vi "DSF.Engine.Transfer Group.Move Channels to Engine.vi"(8 "error in (no error)":errorcluster, 11 "Transfer Group in":refnum<class "DSF.Engine.Transfer Group.lvclass">) -> (0 "error out":errorcluster, 3 "Transfer Group out":refnum<class "DSF.Engine.Transfer Group.lvclass">)   [LabVIEW 2017, in "DSF.Engine.lvlib" / "DSF.Engine.Transfer Group.lvclass"]
uses:
  DSF.Engine.Transfer Group.lvclass
  DSF.Engine.Transfer Group.lvclass/DSF.Engine.Transfer Group.ctl
  DSF.Engine.Transfer.lvclass/DSF.Engine.Transfer.ctl
  DSF.Engine.Transfer.lvclass
  Built/Windows/Dependencies/Memory Manager.lvlibp/1abvi3w/vi.lib/National Instruments/Memory Manager/Classes/Pointer/Memory.Pointer.lvclass
  Pointer/DSF.Engine.Pointer.DBL.lvclass
  C:/Git/DSF/dsf core/Built/Windows/Dependencies/Memory Manager.lvlibp/1abvi3w/vi.lib/National Instruments/Memory Manager/Classes/Pointer/Memory.Pointer.lvclass
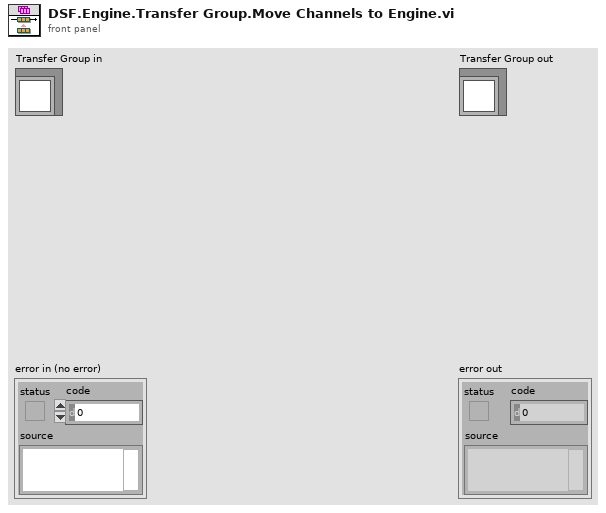
[diagram p1: front panel]
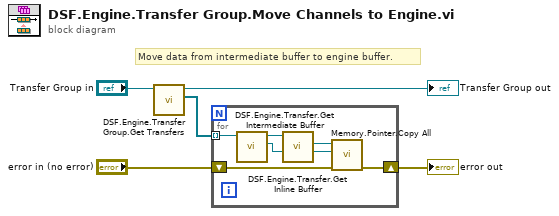
[diagram p0: block diagram]
diagram:
  # "Move data from intermediate buffer to engine buffer."
  n1 = call "DSF.Engine.Transfer Group.Get Transfers.vi"("Transfer Group in"="Transfer Group in") -> ("Transfers"=w4:refnum<class "DSF.Engine.Transfer.lvclass">[], "Transfer Group out"=→"Transfer Group out":refnum<class "DSF.Engine.Transfer Group.lvclass">)  [unwired: 9 in]
  n2 = for {
    tunnel: w4 -> [w9] mode=indexing
    shift-right: [w11] -> w2
    shift-left: "error in (no error)" -> [w10]
    n3 = call "DSF.Engine.Transfer.Get Intermediate Buffer.vi"("Transfer in"=w9) -> ("DBL Buffer"=w8:refnum<class "DSF.Engine.Pointer.DBL.lvclass">, "Transfer out"=w7:refnum<class "DSF.Engine.Transfer.lvclass">)  [unwired: 9 in]
    n4 = call "DSF.Engine.Transfer.Get Inline Buffer.vi"("Transfer in"=w7) -> ("Inline Buffer"=w6:refnum<class "DSF.Engine.Pointer.DBL.lvclass">)  [unwired: 9 in, 1 out]
    n5 = call "Memory.Pointer.Copy All.vi"("error in (no error)"=w10, "dst Pointer in"=w8, "src Pointer in"=w6) -> ("error out"=w11:errorcluster)  [unwired: 6 in, 2 out]
  }
  "error out" <- w2
